vi "buildReplayClusters.vi"(8 "error in (no error)":errorcluster, 11 "Game in":refnum<class "Game.lvclass">) -> (0 "error out":errorcluster, 2 "ReplayInfo":T1, 3 "Game out":refnum<class "Game.lvclass">)   [LabVIEW 2020, in "Game.lvclass"]
uses:
  Game.lvclass
  ReplayInfo.ctl
  RobotExtraInfo.ctl
  Game.lvclass/Game.ctl
  Team_class/Team.lvclass/Team.ctl
  Robot_class/Robot.lvclass/Robot.ctl
  Robot_class/Read id.vi
  Read AllyRef.vi
  Read EnemyRef.vi
  Team_class/Read RobotRef.vi
  Enemy_class/Enemy.lvclass
  C:/Users/anton/Desktop/RoboIME/SSL/SSL_AI/Team_class/Team.lvclass
  Ally_class/Ally.lvclass
  Robot_class/Robot.lvclass
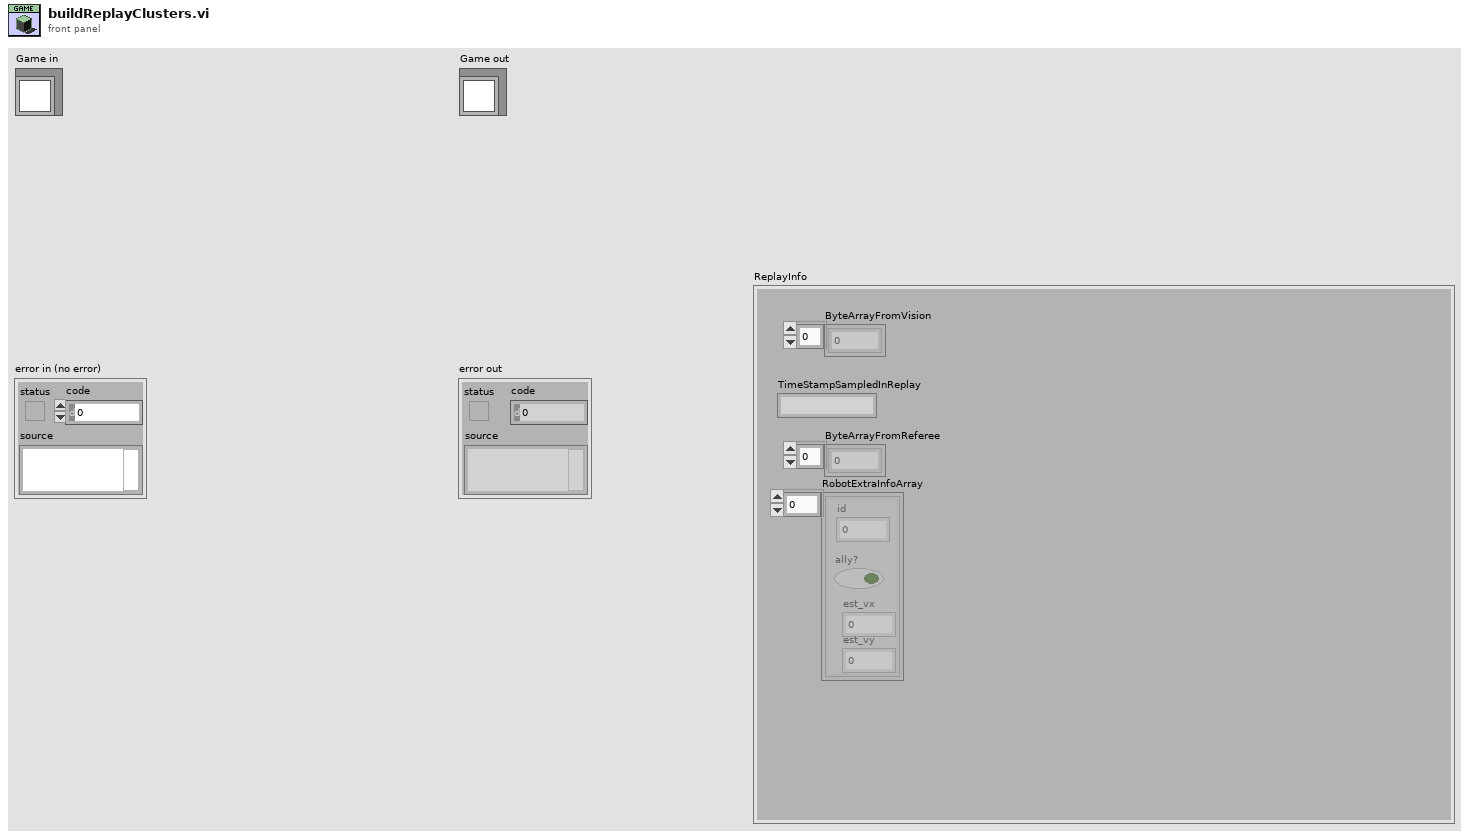
[diagram p1: front panel]
types:
  T1 = typedef "ReplayInfo.ctl" = cluster{"ByteArrayFromVision":u8[], "TimeStampSampledInReplay":string, "ByteArrayFromReferee":u8[], "RobotExtraInfoArray":T2[]}
  T2 = typedef "RobotExtraInfo.ctl" = cluster{"est_vx":dbl, "est_vy":dbl, "id":dbl, "ally?":bool}
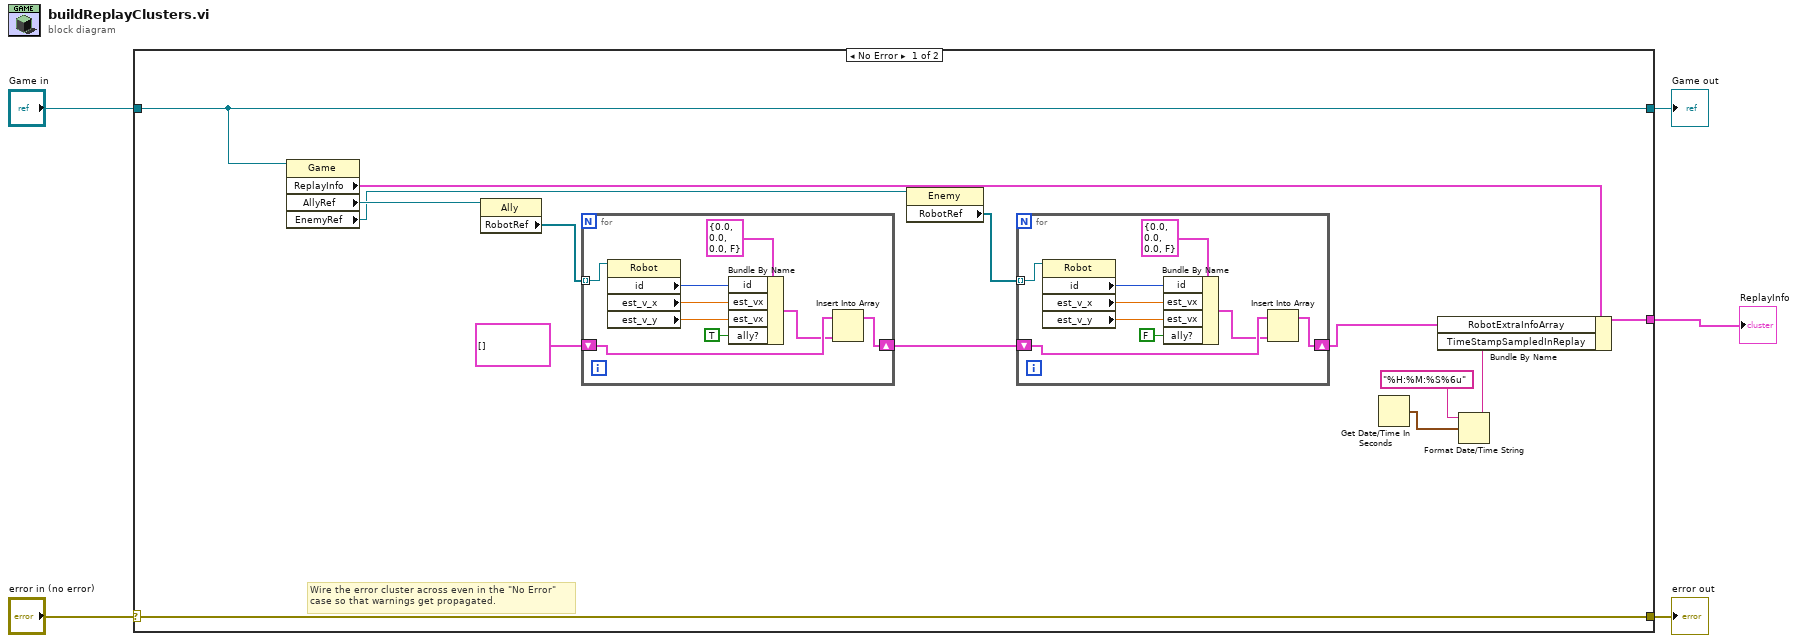
[diagram p0: block diagram]
diagram:
  n1 = case shown="No Error" "error in (no error)" {
    selector: "error in (no error)" -> [w19 w39]
    tunnel: [w19 w39] -> w4
    tunnel: [w18 w38] -> w2
    tunnel: "Game in" -> [w18 w38]
    tunnel: [w17 _] -> w1
    frame No Error {
      # "Wire the error cluster across even in the \"No Error\"\ncase so that warnings get propagated."
      n2 = property class="Game"(reference=w18) -> ("ReplayInfo"=w13:T1, "AllyRef"=w12:refnum<class "Ally.lvclass">, "EnemyRef"=w11:refnum<class "Enemy.lvclass">)  [unwired: 1 in, 2 out]
      n3 = property class="Ally"(reference=w12) -> ("RobotRef"=w10:refnum<class "Robot.lvclass">[])  [unwired: 1 in, 2 out]
      n4 = for {
        tunnel: w10 -> [w37] mode=indexing
        shift-right: [w29] -> w8
        shift-left: T2[] [] ("RobotExtraInfoArray") -> [w31]
        n5 = property class="Robot"(reference=w37) -> ("id"=w35:i32, "est_v_x"=w34:dbl, "est_v_y"=w33:dbl)  [unwired: 1 in, 2 out]
        n6 = Bundle By Name(cluster=T2 {"est_vx"=0.0, "est_vy"=0.0, "id"=0.0, "ally?"=FALSE} ("RobotExtraInfo"), "id"=w35, "est_vx"=w34, "est_vx"=w33, "ally?"=TRUE) -> (w30:T2)
        n7 = Insert Into Array(array=w31, new element=w30) -> (w29:T2[])  [unwired: 1 in]
      }
      n8 = property class="Enemy"(reference=w11) -> ("RobotRef"=w7:refnum<class "Robot.lvclass">[])  [unwired: 1 in, 2 out]
      n9 = for {
        tunnel: w7 -> [w28] mode=indexing
        shift-right: [w20] -> w6
        shift-left: w8 -> [w22]
        n10 = property class="Robot"(reference=w28) -> ("id"=w26:i32, "est_v_x"=w25:dbl, "est_v_y"=w24:dbl)  [unwired: 1 in, 2 out]
        n11 = Bundle By Name(cluster=T2 {"est_vx"=0.0, "est_vy"=0.0, "id"=0.0, "ally?"=FALSE} ("RobotExtraInfo"), "id"=w26, "est_vx"=w25, "est_vx"=w24, "ally?"=FALSE) -> (w21:T2)
        n12 = Insert Into Array(array=w22, new element=w21) -> (w20:T2[])  [unwired: 1 in]
      }
      n13 = Get Date/Time In Seconds() -> (seconds since 1Jan1904=w16:timestamp)
      n14 = Format Date/Time String(time format string (%c)="%H:%M:%S%6u", seconds (now)=w16) -> (date/time string=w14:string)  [unwired: 1 in]
      n15 = Bundle By Name(cluster=w13, "RobotExtraInfoArray"=w6, "TimeStampSampledInReplay"=w14) -> (w17:T1)
    }
    frame Error {
    }
  }
  "error out" <- w4
  "Game out" <- w2
  "ReplayInfo" <- w1
